vi "SetParam.vi"(8 "error in (no error)":errorcluster caption="entrée d'erreur (pas d'erreur)", 10 "TfidfVectorizer":T1={"encoding"="utf-8", "decode_error"="strict", "strip_accents"="None", "lowercase"=TRUE, "preprocessor"="None", "tokenizer"="None", "analyzer"="word", "stop_words"={"Type"="None", "list"=[]}, "token_pattern"="(?u)\\b\\w\\w+\\b", "ngram_range"={"min_n"=1, "max_n"=1}, "max_df"=1.0, "min_df"=1.0, "max_features"=-1, "vocabulary"={"Clé"=["None"], "Valeur"=[]}, "binary"=FALSE, "dtype"="float", "norm"="l2", "use_idf"=TRUE, "smooth_idf"=TRUE, "sublinear_tf"=FALSE} {"max_features" min=-1; "min_df" min=0.0 max=1.0; "max_df" min=0.0 max=1.0}, 11 "TfidfVectorizer.lvclass":refnum<class "TfidfVectorizer.lvclass">) -> (0 "error out":errorcluster caption="sortie d'erreur", 3 "TfidfVectorizer.lvclass":refnum<class "TfidfVectorizer.lvclass">)   [LabVIEW 2020, in "TfidfVectorizer.lvclass"]
doc: "Set Parameters"
uses:
  TfidfVectorizer.lvclass
  TfidfVectorizer.lvclass/TfidfVectorizer.ctl
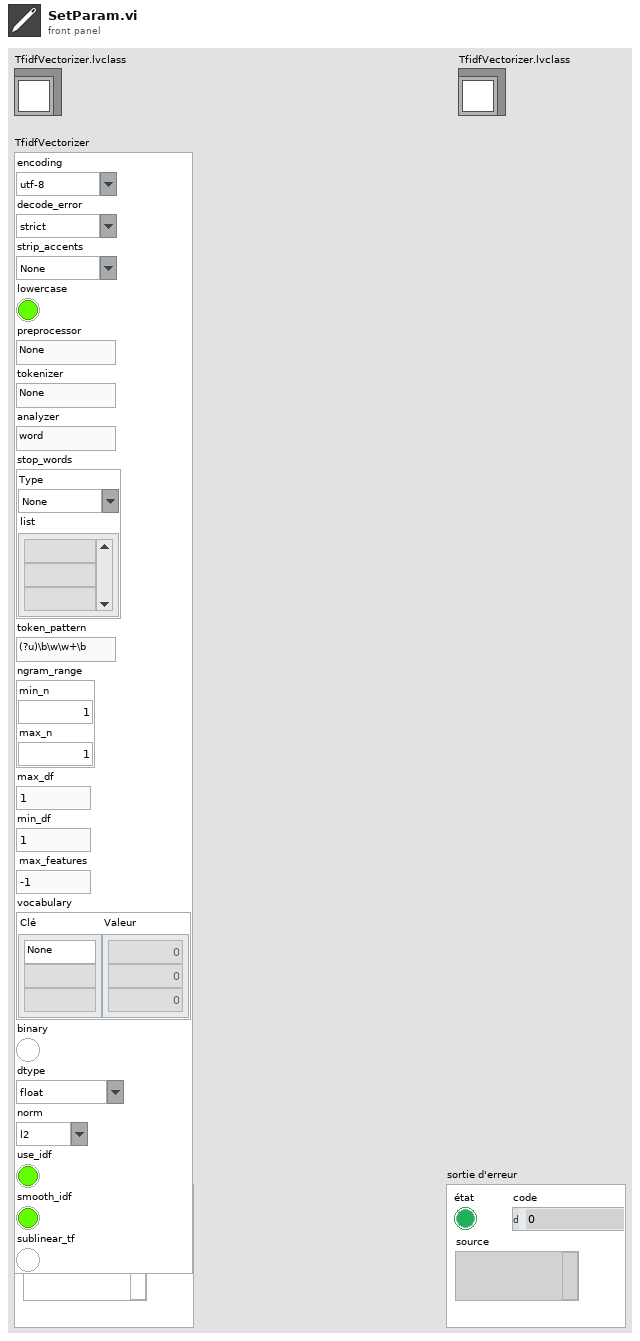
[diagram p1: front panel]
types:
  T1 = cluster{"encoding":string, "decode_error":string, "strip_accents":string, "lowercase":bool, "preprocessor":string, "tokenizer":string, "analyzer":string, "stop_words":cluster{"Type":string, "list":string[]}, "token_pattern":string, "ngram_range":cluster{"min_n":i32, "max_n":i32}, "max_df":dbl, "min_df":dbl, "max_features":i32, "vocabulary":cluster{"Clé":string[], "Valeur":i32[]}, "binary":bool, "dtype":string, "norm":string, "use_idf":bool, "smooth_idf":bool, "sublinear_tf":bool}
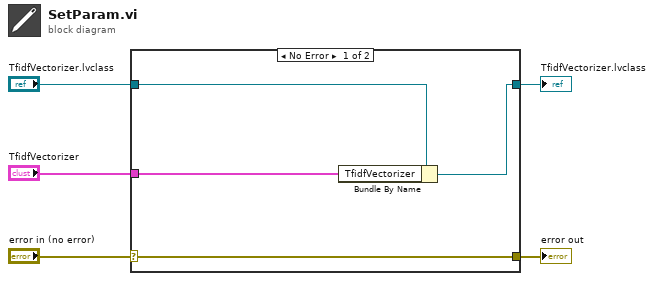
[diagram p0: block diagram]
diagram:
  n1 = case shown="No Error" "error in (no error)" {
    selector: "error in (no error)" -> [w9 w10]
    tunnel: [w9 w10] -> w4
    tunnel: [w7 w11] -> w2
    tunnel: "TfidfVectorizer.lvclass" -> [w8 w11]
    tunnel: "TfidfVectorizer" -> [w6 _]
    frame No Error {
      n2 = Bundle By Name(cluster=w8, "TfidfVectorizer"=w6) -> (w7:refnum<class "TfidfVectorizer.lvclass">)
    }
    frame Error {
    }
  }
  "error out" <- w4
  "TfidfVectorizer.lvclass" <- w2
